vi "Grabber.vi"() -> ()   [LabVIEW 2011]
uses:
  CameraLan.lvclass
  <instrlib>/niHWS/nihws.llb/niHWS Open File Permissions ID.ctl
  <instrlib>/niHWS/nihws.llb/niHWS Write Analog DBL.vi
  <vilib>/userdefined/High Color/IMAQdx.ctl
panel:
  in  "Magnify":bool
  in  "stop":bool
  in  "Compressor":string(combo)="DV Video Encoder"
  in  "quality":i32=-1
  in  "Rec":bool
  in  "Path":path
  in  "Gain":dbl(slide)=1.0 min=1.0 max=3.9810717055349722 scale=1.0..4.0
  out "acquired FPS":dbl
  out "Image":T1(plugin-control)
  in  "Session In":T2="S1019101"
  in  "Fps":i32=60
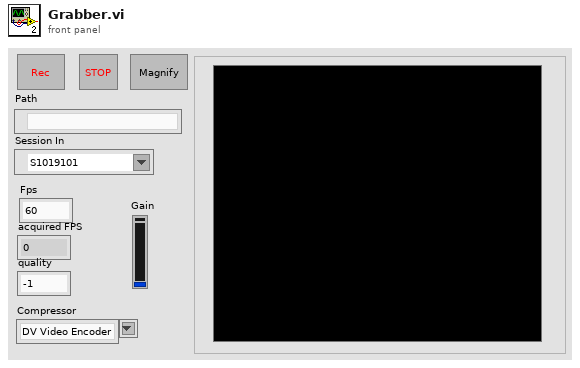
[diagram p1: front panel]
types:
  T1 = typedef "IMAQ Image.ctl" = refnum<image>
  T2 = typedef "IMAQdx.ctl" = refnum<k21>
  T3 = typedef "niHWS Open File Permissions ID.ctl" = enum32{"Read Only", "Read/Write Existing", "Read/Write/Create New", "Read/Write/Create New Always"}
  T4 = typedef "AviRefnum.ctl" = refnum<k1>
  T5 = enum32{"Invalid", "Standard", "Closed", "Hidden", "Minimized", "Maximized"}
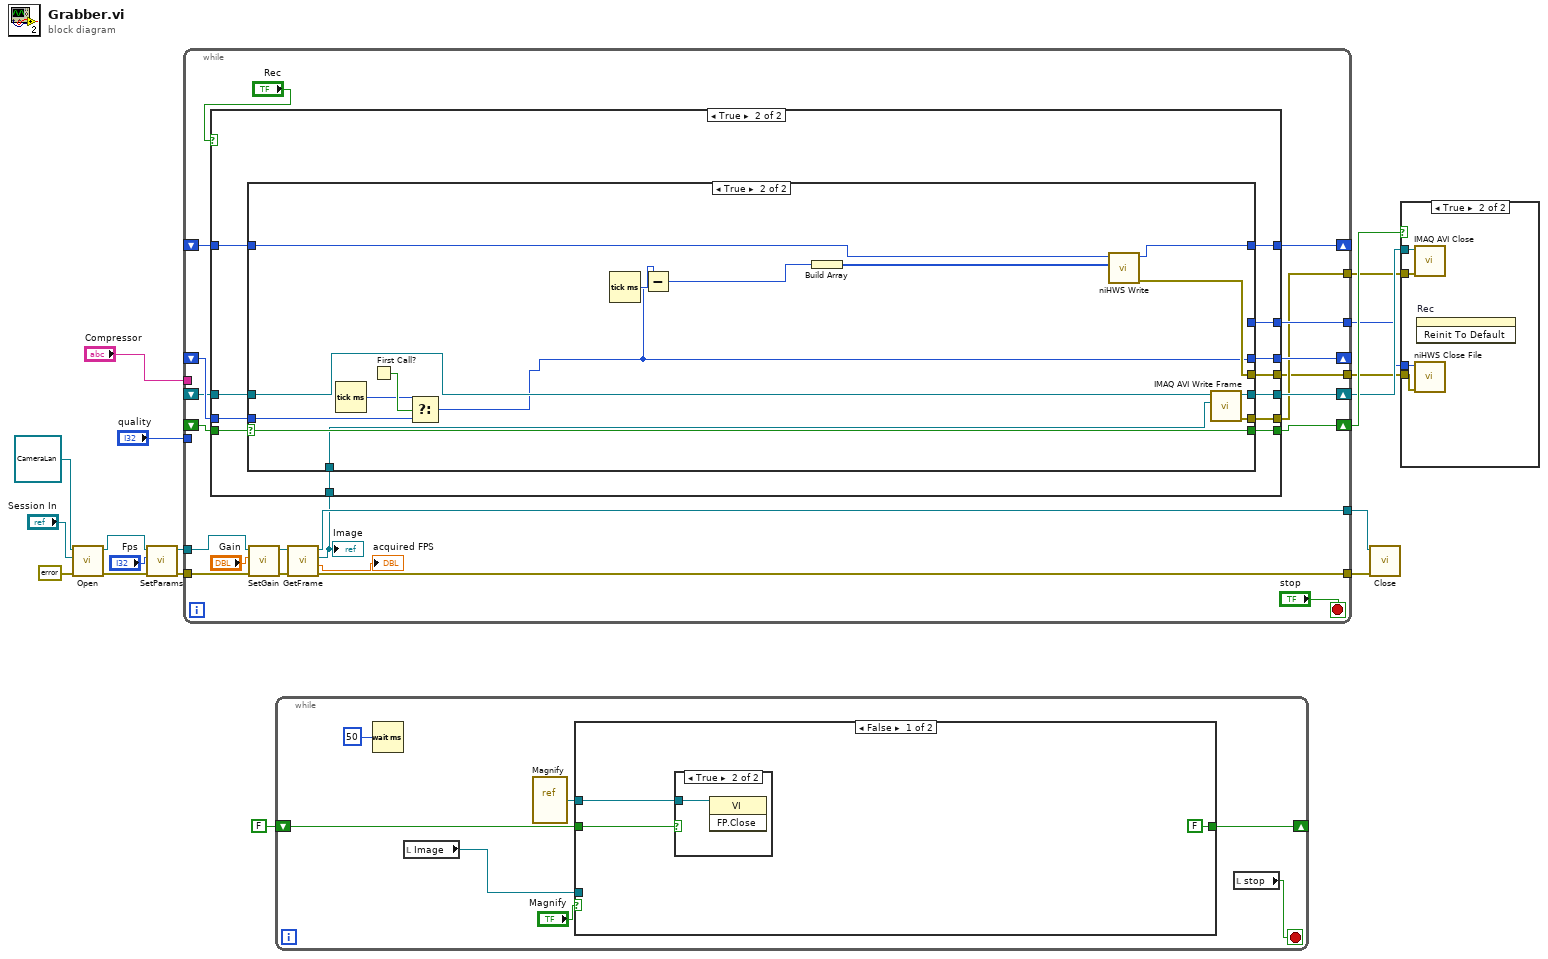
[diagram p0: block diagram]
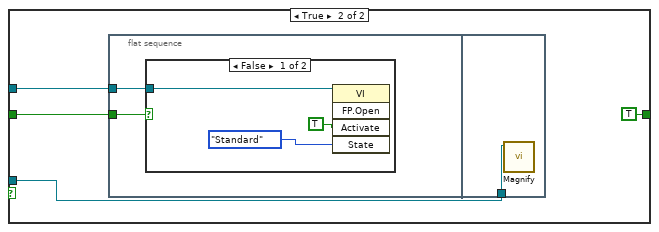
[diagram p3: hidden frame]
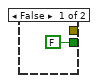
[diagram p6: hidden frame]
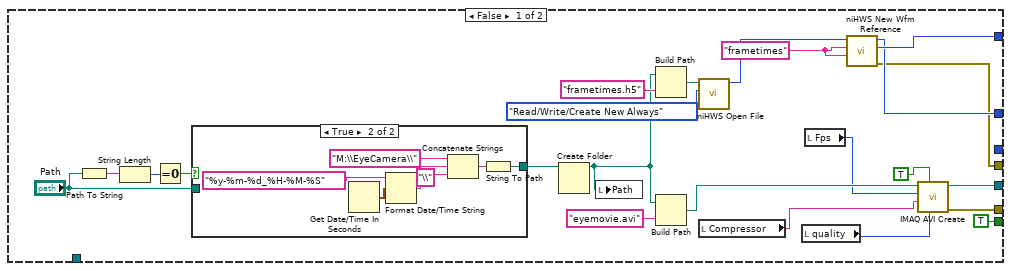
[diagram p7: hidden frame]
diagram:
  n1 = call-dynamic "Open.vi"("error in (no error)"=errorcluster {"status"=FALSE, "code"=0, "source"=""}, "Session In"="Session In", "CameraLan in"=refnum<class "CameraLan.lvclass"> refnum) -> ("error out"=w13:errorcluster, "CameraLan out"=w12:refnum<class "CameraLan.lvclass">)  [unwired: 7 in]
  n2 = call-dynamic "SetParams.vi"("error in (no error)"=w13, "Fps"="Fps", "CameraLan in"=w12) -> ("error out"=w17:errorcluster, "CameraLan out"=w16:refnum<class "CameraLan.lvclass">)  [unwired: 7 in]
  n3 = while {
    tunnel: [w40] -> w15
    tunnel: w16 -> [w38]
    tunnel: w17 -> [w37]
    tunnel: [w35] -> w18
    tunnel: "Compressor" -> [_]
    tunnel: "quality" -> [_]
    shift-right: [w31] -> w6
    shift-left: _ -> [w30]
    shift-right: [w29] -> _
    shift-left: _ -> [w28]
    shift-right: [w27] -> _
    shift-left: _ -> [w26]
    tunnel: [w24] -> w4
    tunnel: [w23] -> w3
    tunnel: [w22] -> w2
    shift-right: [w25] -> w5
    shift-left: _ -> [w19]
    stop <- "stop" stop-if-true
    n4 = call-dynamic "SetGain.vi"("error in (no error)"=w37, "Gain"="Gain", "CameraLan in"=w38) -> ("error out"=w36:errorcluster, "CameraLan out"=w39:refnum<class "CameraLan.lvclass">)  [unwired: 7 in]
    n5 = call-dynamic "GetFrame.vi"("error in (no error)"=w36, "CameraLan in"=w39) -> ("error out"=w35:errorcluster, "acquired FPS"=→"acquired FPS":dbl, "Image Out"=w20:T1, "CameraLan out"=w40:refnum<class "CameraLan.lvclass">)  [unwired: 5 in, 1 out]
    "Image" <- w20
    n6 = case shown="True" "Rec" {
      tunnel: [_ w52] -> w25
      tunnel: [_ w51] -> w23
      tunnel: [FALSE w53] -> w31
      tunnel: [_ w50] -> w27
      tunnel: w30 -> [_ w49]
      tunnel: [_ w48] -> w29
      tunnel: w28 -> [_ w47]
      tunnel: w26 -> [_ w46]
      tunnel: [_ w45] -> w24
      tunnel: [_ w44] -> w22
      tunnel: w20 -> [_ w43]
      tunnel: w19 -> [_ w42]
      frame False {
      }
      frame True {
        n7 = case shown="True" w49 {
          selector: w49 -> [_ w99]
          tunnel: [TRUE w99] -> w53
          tunnel: [w73 w98] -> w52
          tunnel: [w72 w97] -> w51
          tunnel: [w56 w91] -> w50
          tunnel: [_ w85] -> w48
          tunnel: w47 -> [_ w94]
          tunnel: w46 -> [_ w92]
          tunnel: [w55 _] -> w45
          tunnel: [w54 w89] -> w44
          tunnel: w43 -> [_ w88]
          tunnel: w42 -> [_ w87]
          frame False {
            w60 = "frametimes" ("group name (empty)")
            n8 = Path To String(path="Path") -> (string=w74:string)
            n9 = String Length(string=w74) -> (length=w75:i32)
            n10 = Equal To 0?(x=w75) -> (x = 0?=w65:bool)
            n11 = case shown="True" w65 {
              tunnel: [w77 w78] -> w63
              tunnel: "Path" -> [w77 _]
              frame False {
              }
              frame True {
                n12 = Get Date/Time In Seconds() -> (seconds since 1Jan1904=w84:timestamp)
                n13 = Format Date/Time String(time format string (%c)="%y-%m-%d_%H-%M-%S", seconds (now)=w84) -> (date/time string=w81:string)  [unwired: 1 in]
                n14 = Concatenate Strings("M:\\EyeCamera\\", w81, "\\" ("string")) -> (w79:string)
                n15 = String To Path(string=w79) -> (path=w78:path)
              }
            }
            n16 = Create Folder(path (use dialog)=w63) -> (created path=w62:path)  [unwired: 2 in, 2 out]
            n17 = local write "Path"(w62) -> ()
            n18 = Build Path(base path=w62, name or relative path="frametimes.h5" ("search string")) -> (appended path=w66:path)
            n19 = Build Path(base path=w62, name or relative path="eyemovie.avi" ("search string")) -> (appended path=w68:path)
            n20 = call <instrlib>:"niHWS Open File.vi"("permissions (0:read only)"=niHWS_Open_File_Permissions_ID."Read/Write/Create New Always", "file path"=w66) -> ("file handle"=w61:u32)  [unwired: 8 in, 1 out]
            n21 = local read "Compressor"() -> (w58:string)
            n22 = local read "quality"() -> (w57:i32)
            n23 = local read "Fps"() -> (w59:i32)
            n24 = call <instrlib>:"niHWS New Wfm Reference.vi"("waveform name (empty)"=w60, "group name (empty)"=w60, "file handle in"=w61) -> ("error out"=w54:errorcluster, "waveform reference"=w56:u32, "file handle out"=w55:u32)  [unwired: 6 in]
            n25 = call "IMAQ AVI Create"("quality"=w57, "Has Data"=TRUE, "Compression Filter"=w58, "Frames Per Second"=w59, "AVI Path"=w68) -> ("error out"=w72:errorcluster, "Avi Refnum"=w73:T4)  [unwired: 2 in, 3 out]
          }
          frame True {
            n26 = Tick Count (ms)() -> (millisecond timer value=w95:u32)
            n27 = First Call?() -> (First Call?: T/F=w96:bool)
            n28 = Select(t=w95, s=w96, f=w94) -> (s? t:f=w85:u32)
            n29 = Tick Count (ms)() -> (millisecond timer value=w86:u32)
            n30 = Subtract(x=w86, y=w85) -> (x-y=w90:u32)
            n31 = Build Array(w90) -> (w93:u32[])
            n32 = call-poly <instrlib>:"niHWS Write.vi"("data"=w93, "waveform reference in"=w92) -> ("error out"=w89:errorcluster, "waveform reference out"=w91:u32)  [unwired: 8 in]
            n33 = call "IMAQ AVI Write Frame"("Image"=w88, "Avi Refnum"=w87) -> ("error out"=w97:errorcluster, "Avi Refnum (duplicate)"=w98:T4)  [unwired: 8 in]
          }
        }
      }
    }
  }
  n34 = while {
    shift-right: [w104] -> _
    shift-left: FALSE -> [w103]
    stop <- w101 stop-if-true
    n35 = Wait (ms)(milliseconds to wait=u32 50) -> ()  [unwired: 1 out]
    n36 = local read "Image"() -> (w100:T1)
    n37 = vi-ref "Magnify.vi"() -> (w106:refnum<vi>)
    n38 = case shown="False" "Magnify" {
      tunnel: w106 -> [w109 w114]
      tunnel: [FALSE TRUE] -> w104
      tunnel: w103 -> [w108 w112]
      tunnel: w100 -> [_ w111]
      frame False {
        n39 = case shown="True" w108 {
          tunnel: w109 -> [_ w110]
          frame False {
          }
          frame True {
            n40 = invoke class="VI" method="FP.Close"(reference=w110) -> ()  [unwired: 2 in, 3 out]
          }
        }
      }
      frame True {
        n41 = flat-sequence {
          tunnel: w114 -> [w116]
          tunnel: w112 -> [w115]
          tunnel: w111 -> [w120]
          frame #0 {
            n42 = case shown="False" w115 {
              tunnel: w116 -> [w118 _]
              frame False {
                n43 = invoke class="VI" method="FP.Open"(reference=w118, "Activate"=TRUE ("Wait Until Done"), "State"=T5."Standard") -> ()  [unwired: 2 in, 5 out]
              }
              frame True {
              }
            }
          }
          frame #1 {
            n44 = call "Magnify.vi"("Camera 2"=w120) -> ()  [unwired: 11 in]
          }
        }
      }
    }
    n45 = local read "stop"() -> (w101:bool)
  }
  n46 = call-dynamic "Close.vi"("error in (no error)"=w18, "CameraLan in"=w15) -> ()  [unwired: 9 in, 1 out]
  n47 = case shown="True" w6 {
    tunnel: w5 -> [_ w124]
    tunnel: w3 -> [_ w123]
    tunnel: w4 -> [_ w122]
    tunnel: w2 -> [_ w121]
    frame False {
    }
    frame True {
      n48 = call "IMAQ AVI Close"("error in (no error)"=w123, "Avi Refnum"=w124) -> ()  [unwired: 9 in, 1 out]
      n49 = call <instrlib>:"niHWS Close File.vi"("error in (no error)"=w121, "file handle"=w122) -> ()  [unwired: 9 in, 1 out]
      n50 = invoke on="Rec" class="Bool (strict)" method="Reinit To Default"() -> ()  [unwired: 3 in, 3 out]
    }
  }
